vi "Shut Down Device.vi"(8 "error in (no error)":errorcluster, 11 "LQ Laser Quantum in":refnum<class "LQ Laser.lvclass">) -> (0 "error out":errorcluster, 3 "LQ Laser Quantum out":refnum<class "LQ Laser.lvclass">)   [LabVIEW 2023, in "LQ Laser.lvlib" / "LQ Laser.lvclass"]
uses:
  LQ Laser.lvclass
  LQ Laser.lvclass/LQ Laser.ctl
  Laser/Laser.lvclass
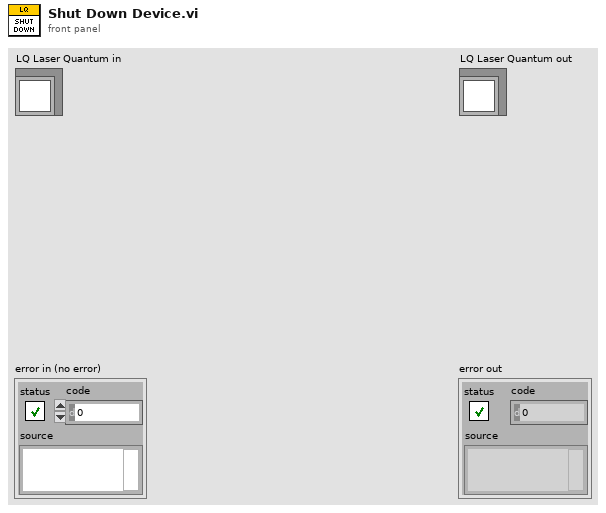
[diagram p1: front panel]
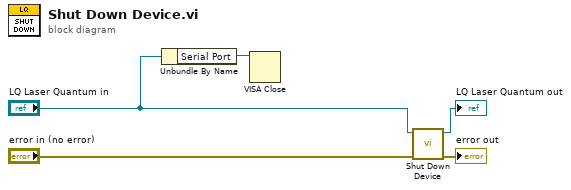
[diagram p0: block diagram]
diagram:
  n1 = Unbundle By Name("LQ Laser Quantum in") -> ("Serial Port"=w2:refnum<visa-resource-name>)
  n2 = VISA Close(VISA resource name=w2) -> ()  [unwired: 1 in, 1 out]
  n3 = call-parent "Shut Down Device.vi"("error in (no error)"="error in (no error)", "Device in"="LQ Laser Quantum in") -> ("error out"=→"error out":errorcluster, "Device out"=→"LQ Laser Quantum out":refnum<class "LQ Laser.lvclass">)  [unwired: 8 in]
